vi "Register gRPC Messages.vi"(8 "error in (no error)":errorcluster, 11 "gRPC ID":T1) -> (0 "error out":errorcluster, 3 "gRPC ID Out":T1)   [LabVIEW 2019, in "Generated_server.lvlib"]
uses:
  Generated_server.lvlib
  <vilib>/gRPC/LabVIEW gRPC Library/Shared/grpcId.ctl
  <vilib>/gRPC/LabVIEW gRPC Library/Server API/typeDefs/Message Metadata.ctl
  <vilib>/gRPC/LabVIEW gRPC Library/Server API/typeDefs/Message Element Metadata.ctl
  <vilib>/gRPC/LabVIEW gRPC Library/Server API/typeDefs/Message Element Type.ctl
  <vilib>/gRPC/LabVIEW gRPC Library/Server API/typeDefs/Enum Metadata.ctl
  <vilib>/gRPC/LabVIEW gRPC Library/grpc-lvsupport-release.lvlib
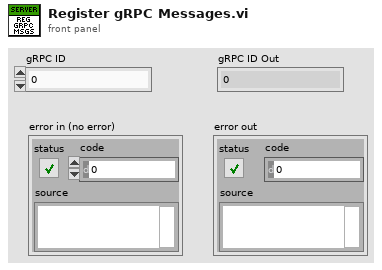
[diagram p1: front panel]
types:
  T1 = typedef "grpc-lvsupport-release.lvlib/grpcId.ctl" = u64
  T2 = typedef "grpc-lvsupport-release.lvlib/Enum Metadata.ctl" = cluster{"Version":i32, "Name":string, "Type Url":string, "Enum Values":string, "Allow Alias":bool}
  T3 = typedef "grpc-lvsupport-release.lvlib/Message Metadata.ctl" = cluster{"Version":i32, "Name":string, "Type Url":string, "Elements":T4[], "Has Oneof":bool}
  T4 = typedef "grpc-lvsupport-release.lvlib/Message Element Metadata.ctl" = cluster{"Field Name":string, "Embedded Message Name":string, "Protobuf Index":i32, "MessageElementType":T5, "Repeated":bool, "Is in Oneof":bool, "Oneof Container Name":string}
  T5 = typedef "grpc-lvsupport-release.lvlib/Message Element Type.ctl" = enum32{"Int32Value", "FloatValue", "DoubleValue", "BoolValue", "StringValue", "MessageValue", "Int64Value", "UInt32Value", "UInt64Value", "EnumValue", "Bytes", "Fixed64", "Fixed32", "SFixed64", "SFixed32", "SInt64", "SInt32"}
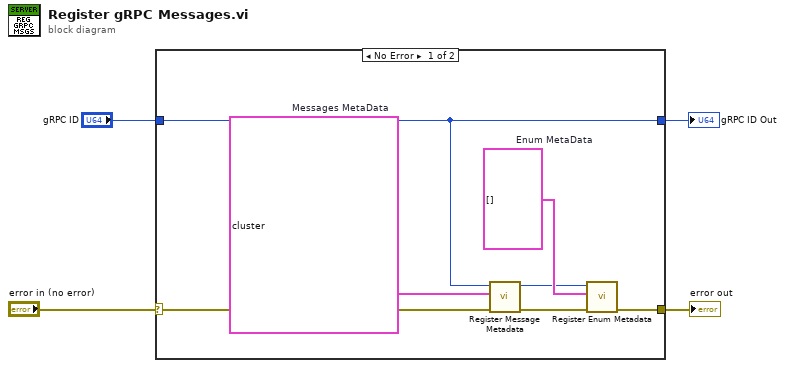
[diagram p0: block diagram]
diagram:
  n1 = case shown="No Error" "error in (no error)" {
    selector: "error in (no error)" -> [w10 w13]
    tunnel: [w9 w12] -> w1
    tunnel: [w5 w13] -> w4
    tunnel: "gRPC ID" -> [w9 w12]
    frame No Error {
      w8 = T2[] []  # Enum MetaData
      w11 = T3[] [{"Version"=2, "Name"="Greeter_res", "Type Url"="Greeter.res", "Elements"=[{"Field Name"="res_latitude", "Embedded Message Name"="", "Protobuf Index"=1, "MessageElementType"=enum."Int32Value", "Repeated"=FALSE, "Is in Oneof"=FALSE, "Oneof Container Name"=""}, {"Field Name"="selected_index", "Embedded Message Name"="", "Protobuf Index"=-1, "MessageElementType"=enum."Int32Value", "Repeated"=FALSE, "Is in Oneof"=TRUE, "Oneof Container Name"="Greeter_res_res_oneof"}, {"Field Name"="res_int32", "Embedded Message Name"="", "Protobuf Index"=2, "MessageElementType"=enum."Int32Value", "Repeated"=FALSE, "Is in Oneof"=TRUE, "Oneof Container Name"="Greeter_res_res_oneof"}, {"Field Name"="res_int64", "Embedded Message Name"="", "Protobuf Index"=3, "MessageElementType"=enum."Int64Value", "Repeated"=FALSE, "Is in Oneof"=TRUE, "Oneof Container Name"="Greeter_res_res_oneof"}, {"Field Name"="res_uint32", "Embedded Message Name"="", "Protobuf Index"=4, "MessageElementType"=enum."UInt32Value", "Repeated"=FALSE, "Is in Oneof"=TRUE, "Oneof Container Name"="Greeter_res_res_oneof"}, {"Field Name"="res_uint64", "Embedded Message Name"="", "Protobuf Index"=5, "MessageElementType"=enum."UInt64Value", "Repeated"=FALSE, "Is in Oneof"=TRUE, "Oneof Container Name"="Greeter_res_res_oneof"}, {"Field Name"="res_sint32", "Embedded Message Name"="", "Protobuf Index"=6, "MessageElementType"=enum."SInt32", "Repeated"=FALSE, "Is in Oneof"=TRUE, "Oneof Container Name"="Greeter_res_res_oneof"}, {"Field Name"="res_sint64", "Embedded Message Name"="", "Protobuf Index"=7, "MessageElementType"=enum."SInt64", "Repeated"=FALSE, "Is in Oneof"=TRUE, "Oneof Container Name"="Greeter_res_res_oneof"}, {"Field Name"="res_fixed32", "Embedded Message Name"="", "Protobuf Index"=8, "MessageElementType"=enum."Fixed32", "Repeated"=FALSE, "Is in Oneof"=TRUE, "Oneof Container Name"="Greeter_res_res_oneof"}, {"Field Name"="res_fixed64", "Embedded Message Name"="", "Protobuf Index"=9, "MessageElementType"=enum."Fixed64", "Repeated"=FALSE, "Is in Oneof"=TRUE, "Oneof Container Name"="Greeter_res_res_oneof"}, {"Field Name"="res_sfixed32", "Embedded Message Name"="", "Protobuf Index"=10, "MessageElementType"=enum."SFixed32", "Repeated"=FALSE, "Is in Oneof"=TRUE, "Oneof Container Name"="Greeter_res_res_oneof"}, {"Field Name"="res_sfixed64", "Embedded Message Name"="", "Protobuf Index"=11, "MessageElementType"=enum."SFixed64", "Repeated"=FALSE, "Is in Oneof"=TRUE, "Oneof Container Name"="Greeter_res_res_oneof"}, {"Field Name"="res_float", "Embedded Message Name"="", "Protobuf Index"=12, "MessageElementType"=enum."FloatValue", "Repeated"=FALSE, "Is in Oneof"=TRUE, "Oneof Container Name"="Greeter_res_res_oneof"}, {"Field Name"="res_double", "Embedded Message Name"="", "Protobuf Index"=13, "MessageElementType"=enum."DoubleValue", "Repeated"=FALSE, "Is in Oneof"=TRUE, "Oneof Container Name"="Greeter_res_res_oneof"}, {"Field Name"="res_bool", "Embedded Message Name"="", "Protobuf Index"=14, "MessageElementType"=enum."BoolValue", "Repeated"=FALSE, "Is in Oneof"=TRUE, "Oneof Container Name"="Greeter_res_res_oneof"}, {"Field Name"="res_string", "Embedded Message Name"="", "Protobuf Index"=15, "MessageElementType"=enum."StringValue", "Repeated"=FALSE, "Is in Oneof"=TRUE, "Oneof Container Name"="Greeter_res_res_oneof"}, {"Field Name"="res_bytes", "Embedded Message Name"="", "Protobuf Index"=16, "MessageElementType"=enum."Bytes", "Repeated"=FALSE, "Is in Oneof"=TRUE, "Oneof Container Name"="Greeter_res_res_oneof"}], "Has Oneof"=TRUE}, {"Version"=2, "Name"="Greeter_req", "Type Url"="Greeter.req", "Elements"=[{"Field Name"="req_latitude", "Embedded Message Name"="", "Protobuf Index"=1, "MessageElementType"=enum."Int32Value", "Repeated"=FALSE, "Is in Oneof"=FALSE, "Oneof Container Name"=""}, {"Field Name"="selected_index", "Embedded Message Name"="", "Protobuf Index"=-1, "MessageElementType"=enum."Int32Value", "Repeated"=FALSE, "Is in Oneof"=TRUE, "Oneof Container Name"="Greeter_req_req_oneof"}, {"Field Name"="req_int32", "Embedded Message Name"="", "Protobuf Index"=2, "MessageElementType"=enum."Int32Value", "Repeated"=FALSE, "Is in Oneof"=TRUE, "Oneof Container Name"="Greeter_req_req_oneof"}, {"Field Name"="req_int64", "Embedded Message Name"="", "Protobuf Index"=3, "MessageElementType"=enum."Int64Value", "Repeated"=FALSE, "Is in Oneof"=TRUE, "Oneof Container Name"="Greeter_req_req_oneof"}, {"Field Name"="req_uint32", "Embedded Message Name"="", "Protobuf Index"=4, "MessageElementType"=enum."UInt32Value", "Repeated"=FALSE, "Is in Oneof"=TRUE, "Oneof Container Name"="Greeter_req_req_oneof"}, {"Field Name"="req_uint64", "Embedded Message Name"="", "Protobuf Index"=5, "MessageElementType"=enum."UInt64Value", "Repeated"=FALSE, "Is in Oneof"=TRUE, "Oneof Container Name"="Greeter_req_req_oneof"}, {"Field Name"="req_sint32", "Embedded Message Name"="", "Protobuf Index"=6, "MessageElementType"=enum."SInt32", "Repeated"=FALSE, "Is in Oneof"=TRUE, "Oneof Container Name"="Greeter_req_req_oneof"}, {"Field Name"="req_sint64", "Embedded Message Name"="", "Protobuf Index"=7, "MessageElementType"=enum."SInt64", "Repeated"=FALSE, "Is in Oneof"=TRUE, "Oneof Container Name"="Greeter_req_req_oneof"}, {"Field Name"="req_fixed32", "Embedded Message Name"="", "Protobuf Index"=8, "MessageElementType"=enum."Fixed32", "Repeated"=FALSE, "Is in Oneof"=TRUE, "Oneof Container Name"="Greeter_req_req_oneof"}, {"Field Name"="req_fixed64", "Embedded Message Name"="", "Protobuf Index"=9, "MessageElementType"=enum."Fixed64", "Repeated"=FALSE, "Is in Oneof"=TRUE, "Oneof Container Name"="Greeter_req_req_oneof"}, {"Field Name"="req_sfixed32", "Embedded Message Name"="", "Protobuf Index"=10, "MessageElementType"=enum."SFixed32", "Repeated"=FALSE, "Is in Oneof"=TRUE, "Oneof Container Name"="Greeter_req_req_oneof"}, {"Field Name"="req_sfixed64", "Embedded Message Name"="", "Protobuf Index"=11, "MessageElementType"=enum."SFixed64", "Repeated"=FALSE, "Is in Oneof"=TRUE, "Oneof Container Name"="Greeter_req_req_oneof"}, {"Field Name"="req_float", "Embedded Message Name"="", "Protobuf Index"=12, "MessageElementType"=enum."FloatValue", "Repeated"=FALSE, "Is in Oneof"=TRUE, "Oneof Container Name"="Greeter_req_req_oneof"}, {"Field Name"="req_double", "Embedded Message Name"="", "Protobuf Index"=13, "MessageElementType"=enum."DoubleValue", "Repeated"=FALSE, "Is in Oneof"=TRUE, "Oneof Container Name"="Greeter_req_req_oneof"}, {"Field Name"="req_bool", "Embedded Message Name"="", "Protobuf Index"=14, "MessageElementType"=enum."BoolValue", "Repeated"=FALSE, "Is in Oneof"=TRUE, "Oneof Container Name"="Greeter_req_req_oneof"}, {"Field Name"="req_string", "Embedded Message Name"="", "Protobuf Index"=15, "MessageElementType"=enum."StringValue", "Repeated"=FALSE, "Is in Oneof"=TRUE, "Oneof Container Name"="Greeter_req_req_oneof"}, {"Field Name"="req_bytes", "Embedded Message Name"="", "Protobuf Index"=16, "MessageElementType"=enum."Bytes", "Repeated"=FALSE, "Is in Oneof"=TRUE, "Oneof Container Name"="Greeter_req_req_oneof"}], "Has Oneof"=TRUE}]  # Messages MetaData
      n2 = call <vilib>:"Register Message Metadata.vi"("error in"=w10, "Messages"=w11, "gRPCid in"=w9) -> ("error out"=w6:errorcluster, "gRPCid out"=w7:T1)  [unwired: 7 in]
      n3 = call <vilib>:"Register Enum Metadata.vi"("error in"=w6, "Enum Metadata"=w8, "gRPCid in"=w7) -> ("error out"=w5:errorcluster)  [unwired: 7 in, 1 out]
    }
    frame Error {
    }
  }
  "error out" <- w4
  "gRPC ID Out" <- w1
